vi "ConnectCamera.vi"() -> (0 "error out":errorcluster, 1 "params":variant, 2 "port":u16, 3 "camera":refnum<class "CameraBase.lvclass">, 4 "camera name":string, 5 "zlock":string, 7 "conn table":path)   [LabVIEW 2010]
uses:
  <userlib>/bias/classes/CameraBase/CameraBase.lvclass
  <userlib>/_OpenG.lib/array/array.llb/Search 1D Array (Boolean)__ogtk.vi
  <userlib>/_OpenG.lib/error/error.llb/Filter Error Codes (Array)__ogtk.vi
  <vilib>/addons/h5labview2/file/H5F.lvlib
  <vilib>/addons/h5labview2/attrib/H5A.lvlib
panel:
  in  "offline":bool
  in  "cancel":bool
  in  "connect":bool
  in  "cameras":i32(listbox)
  # "Select camera to connect to:"
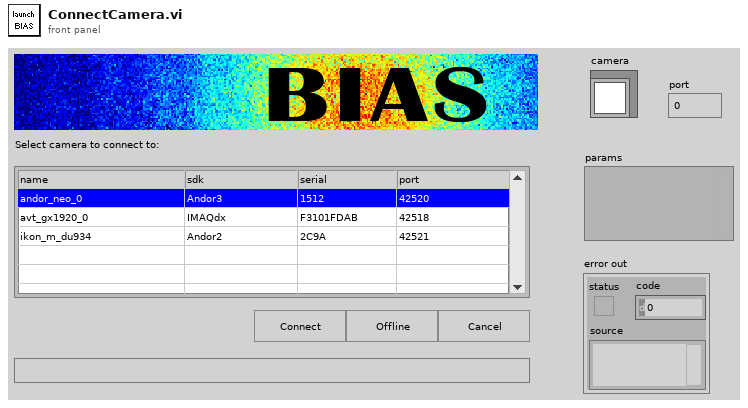
[diagram p1: front panel]
types:
  T1 = typedef "CameraInfo.ctl" = cluster{"name":string, "serial":u64, "interface":string, "make":string, "model":string, "pixel_w":dbl, "pixel_h":dbl}
  T2 = typedef "hid_t.ctl" = i32
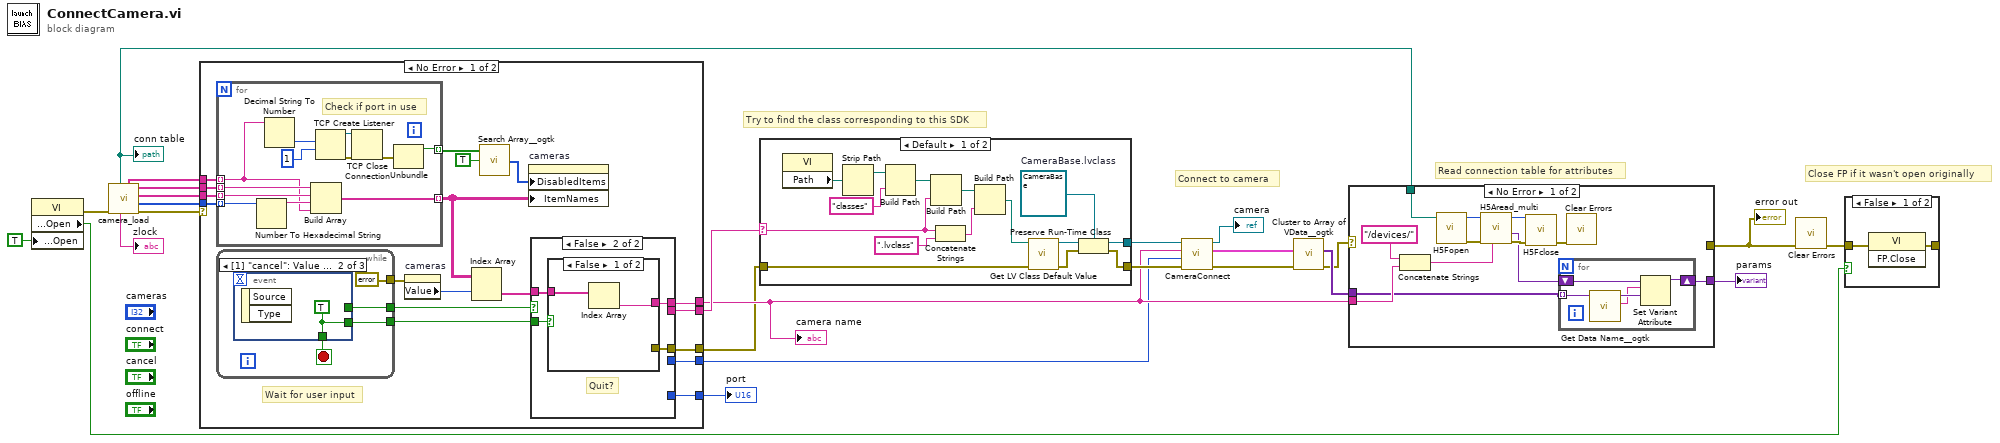
[diagram p0: block diagram]
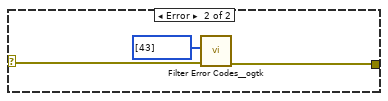
[diagram p4: hidden frame]
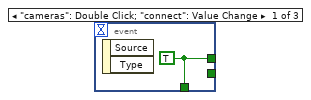
[diagram p5: hidden frame]
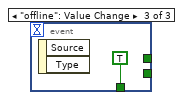
[diagram p6: hidden frame]
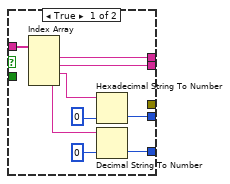
[diagram p7: hidden frame]
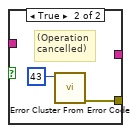
[diagram p8: hidden frame]
diagram:
  # "Close FP if it wasn't open originally"
  # "Connect to camera"
  # "Try to find the class corresponding to this SDK"
  # "Read connection table for attributes"
  n1 = property class="VI"("Front Panel.Open"=TRUE ("Front Panel Window:Open")) -> (error out=w7:errorcluster, "Front Panel.Open"=w3:bool)  [unwired: 2 in, 1 out]
  n2 = call <userlib>:"camera_load.vi"("error in (no error)"=w7) -> ("error out"=w19:errorcluster, "serials"=w25:u64[], "sdks"=w24:string[], "names"=w23:string[], "ports"=w22:string[], "zlock"=→"zlock":string, "hdf"=w21:path)  [unwired: 3 in]
  "conn table" <- w21
  n3 = case shown="No Error" w19 {
    selector: w19 -> [_ w80]
    tunnel: [w43 w80] -> w11
    tunnel: w25 -> [w42 _]
    tunnel: w24 -> [w41 _]
    tunnel: w23 -> [w40 _]
    tunnel: w22 -> [w39 _]
    tunnel: [w38 _] -> w20
    tunnel: [w37 _] -> w13
    tunnel: [w32 _] -> w16
    tunnel: [w31 _] -> w12
    frame No Error {
      # "Wait for user input"
      n4 = for {
        tunnel: w40 -> [w62] mode=indexing
        tunnel: w41 -> [w61] mode=indexing
        tunnel: w42 -> [w60] mode=indexing
        tunnel: [w58] -> w30 mode=indexing
        tunnel: w39 -> [w57] mode=indexing
        tunnel: [w51] -> w36 mode=indexing
        # "Check if port in use"
        n5 = Number To Hexadecimal String(2:w60) -> (0:w59:string)  [unwired: 1 in]
        n6 = Decimal String To Number(string=w57) -> (number=w56:i32)  [unwired: 2 in, 1 out]
        n7 = Build Array(w62, w61, w59, w57) -> (w58:string[])
        n8 = TCP Create Listener(9:1 ("timeout ms (25000)"), 10:w56) -> (0:w54:errorcluster, 3:w53:refnum<k5>)  [unwired: 3 in, 1 out]
        n9 = TCP Close Connection(connection ID=w53, error in (no error)=w54) -> (error out=w52:errorcluster)  [unwired: 1 in, 1 out]
        n10 = Unbundle(w52) -> ("status"=w51:bool)  [unwired: 2 out]
      }
      n11 = while {
        tunnel: [w47] -> w28
        tunnel: [w45] -> w33
        tunnel: [errorcluster {"status"=FALSE, "code"=0, "source"=""} ("error IO")] -> w26
        stop <- w46 stop-if-true
        n12 = event shown="[1] \"cancel\": Value Change;  Panel Close" {
          selector: _ -> [_ _ _]
          dyn-events: _ -> [_ _ _]
          timeout: _ -> [_ _ _]
          tunnel: [w48 _ _] -> w47
          tunnel: [w48 w49 TRUE ("ok")] -> w46
          tunnel: [_ w49 _] -> w45
          event "cameras": Double Click; "connect": Value Change {
            w48 = TRUE ("ok")
            n13 = event-data() -> ()  [unwired: 1 in, 2 out]
          }
          event "cancel": Value Change; Panel Close {
            w49 = TRUE ("ok")
            n14 = event-data() -> ()  [unwired: 1 in, 2 out]
          }
          event "offline": Value Change {
            n15 = event-data() -> ()  [unwired: 1 in, 2 out]
          }
        }
      }
      n16 = property on="cameras" class="MCListbox (strict)"(error in=w26) -> ("Value"=w27:i32)  [unwired: 1 in, 2 out]
      n17 = Index Array(array=w30, index (row)=w27) -> (element=w29:string[])  [unwired: 1 in]
      n18 = call-poly <userlib>:"Search Array__ogtk.vi"("Array"=w36, "Element Data"=TRUE) -> ("Indices of Elements"=w34:i32[])  [unwired: 7 in]
      n19 = property on="cameras" class="MCListbox (strict)"("DisabledItems"=w34, "ItemNames"=w30) -> ()  [unwired: 2 in, 2 out]
      n20 = case shown="False" w28 {
        tunnel: [_ w75] -> w43
        tunnel: [w66 w72] -> w37
        tunnel: [w69 _] -> w38
        tunnel: w33 -> [_ w74]
        tunnel: [w65 _] -> w32
        tunnel: [w64 _] -> w31
        tunnel: w29 -> [w63 w73]
        frame True {
          n21 = Index Array(array=w63) -> (element #1=w66:string, element #2=w65:string, element #3=w68:string, element #4=w70:string)  [unwired: 4 in]
          n22 = Hexadecimal String To Number(string=w68, default (0uL)=u64 0 ("default (0 U32)")) -> (number=w64:u64)  [unwired: 1 in, 1 out]
          n23 = Decimal String To Number(string=w70, default (0L)=u16 0 ("default (0 I32)")) -> (number=w69:u16)  [unwired: 1 in, 1 out]
        }
        frame False {
          # "Quit?"
          n24 = case shown="False" w74 {
            tunnel: [_ w79] -> w75
            tunnel: w73 -> [w77 _]
            tunnel: [w76 _] -> w72
            frame False {
              n25 = Index Array(array=w77) -> (element=w76:string)  [unwired: 1 in]
            }
            frame True {
              # "(Operation\ncancelled)"
              n26 = call <vilib>:"Error Cluster From Error Code.vi"("error code (0)"=43) -> ("error out"=w79:errorcluster)  [unwired: 8 in]
            }
          }
        }
      }
    }
    frame Error {
    }
  }
  "port" <- w20
  "camera name" <- w13
  n27 = case shown="Default" w16 {
    selector: w16 -> [w89 _]
    tunnel: [w85 _] -> w15
    tunnel: w11 -> [w83 w96]
    tunnel: [w82 w96] -> w14
    frame Default {
      w81 = refnum<class "CameraBase.lvclass"> refnum  # CameraBase.lvclass
      n28 = property on="Property Node" class="VI"() -> ("Path"=w95:path)  [unwired: 2 in, 2 out]
      n29 = Strip Path(path=w95) -> (stripped path=w94:path)  [unwired: 1 out]
      n30 = Build Path(base path=w94, name or relative path="classes") -> (appended path=w92:path)
      n31 = Build Path(base path=w92, name or relative path=w89) -> (appended path=w91:path)
      n32 = Concatenate Strings(w89, ".lvclass" ("string")) -> (w88:string)
      n33 = Build Path(base path=w91, name or relative path=w88) -> (appended path=w90:path)
      n34 = call <vilib>:"Get LV Class Default Value.vi"("error in (no error)"=w83, "class path"=w90) -> ("error out"=w84:errorcluster, "object"=w86:refnum<class>)  [unwired: 8 in]
      n35 = Preserve Run-Time Class(object in=w86, error in=w84, 2:w81) -> (object out=w85:refnum<class "CameraBase.lvclass">, error out=w82:errorcluster)
    }
    frame "" {
      # "Cancelled OR offline"
    }
  }
  n36 = call-dynamic "CameraConnect.vi"("error in (no error)"=w14, "serial"=w12, "name"=w13, "CameraBase in"=w15) -> ("error out"=w2:errorcluster, "CameraInfo"=w10:T1, "CameraBase out"=→"camera":refnum<class "CameraBase.lvclass">)  [unwired: 5 in]
  n37 = call <userlib>:"Cluster to Array of VData__ogtk.vi"("error in (no error)"=w2, "Cluster"=w10) -> ("error out"=w8:errorcluster, "Array of VData"=w9:variant[])  [unwired: 8 in]
  n38 = case shown="No Error" w8 {
    selector: w8 -> [_ w116]
    tunnel: w21 -> [w105 _]
    tunnel: w13 -> [w107 _]
    tunnel: [_ w115] -> w6
    tunnel: [w106 _] -> w18
    tunnel: w9 -> [w97 _]
    frame No Error {
      n39 = Concatenate Strings("/devices/", w107) -> (w101:string)
      n40 = call <vilib>:"H5Fopen.vi"("path"=w105) -> ("error out"=w100:errorcluster, "ref out"=w103:T2)  [unwired: 9 in]
      n41 = call <vilib>:"H5Aread_multi.vi"("object name"=w101, "error in (no error)"=w100, "ref in"=w103) -> ("error out"=w99:errorcluster, "attribs out"=w98:variant, "ref out"=w102:T2)  [unwired: 5 in, 1 out]
      n42 = call <vilib>:"H5Fclose.vi"("error in (no error)"=w99, "ref"=w102) -> ("error out"=w104:errorcluster)  [unwired: 9 in]
      n43 = for {
        tunnel: w97 -> [w111] mode=indexing
        shift-right: [w110] -> w106
        shift-left: w98 -> [w109]
        n44 = call <userlib>:"Get Data Name__ogtk.vi"("Data"=w111) -> ("Data Name"=w112:string, "Data dup"=w113:variant)  [unwired: 8 in, 1 out]
        n45 = Set Variant Attribute(Variant=w109, name=w112, value=w113) -> (Variant out=w110:variant)  [unwired: 1 in, 2 out]
      }
      n46 = call <vilib>:"Clear Errors.vi"("error in (no error)"=w104) -> ()  [unwired: 6 in, 1 out]
    }
    frame Error {
      n47 = call-poly <userlib>:"Filter Error Codes__ogtk.vi"("Error In"=w116, "Error Codes to Filter"=i32[] [43]) -> ("Error Out"=w115:errorcluster)  [unwired: 7 in, 2 out]
    }
  }
  "params" <- w18
  "error out" <- w6
  n48 = call <vilib>:"Clear Errors.vi"("error in (no error)"=w6) -> ("error out"=w5:errorcluster)  [unwired: 6 in]
  n49 = case shown="False" w3 {
    tunnel: w5 -> [w118 _]
    tunnel: [w117 _] -> _
    frame False {
      n50 = invoke class="VI" method="FP.Close"(error in=w118) -> (error out=w117:errorcluster)  [unwired: 2 in, 2 out]
    }
    frame True {
    }
  }
